vi "test Log Archive.vi"(8 "error in (no error)":errorcluster, 11 "TestCase in":refnum<class "Embedded Data Logger Windows System Tests.lvclass">) -> (0 "error out":errorcluster, 3 "TestCase out":refnum<class "Embedded Data Logger Windows System Tests.lvclass">)   [LabVIEW 2027, in "Embedded Data Logger Windows System Tests.lvclass"]
uses:
  Embedded Data Logger Windows System Tests.lvclass
  61a2513e-13d3-4fa2-bc23-ec2f6314a367.vi
  C:/Program Files/National Instruments/LabVIEW 2027/vi.lib/addons/_JKI Toolkits/VI Tester/TestCase.llb/TestCase.lvclass
  <vilib>/addons/_JKI Toolkits/VI Tester/TestCase.llb/TestCase.lvclass
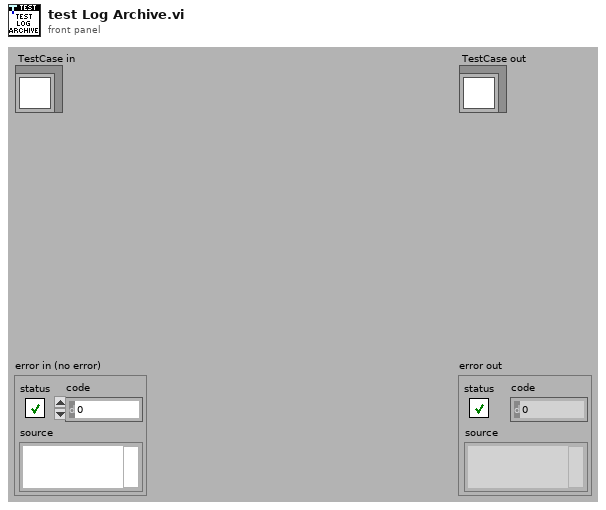
[diagram p1: front panel]
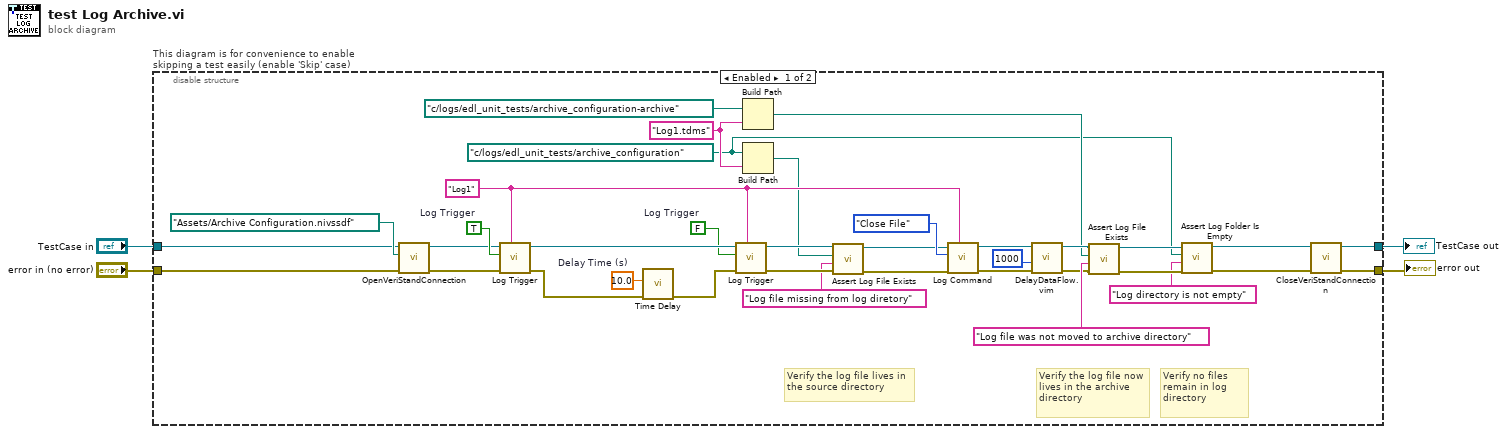
[diagram p0: block diagram]
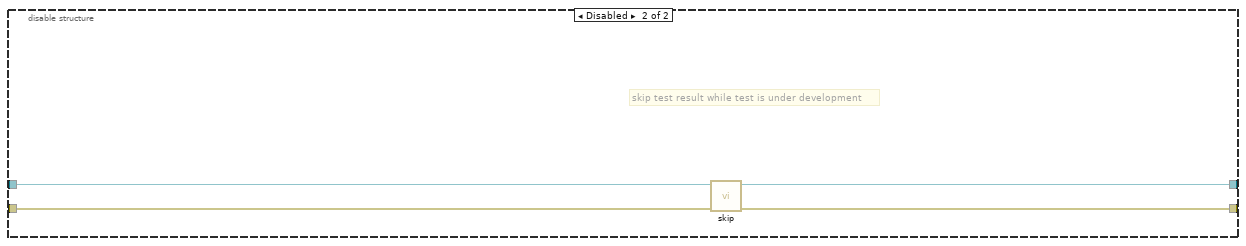
[diagram p2: hidden frame]
diagram:
  n1 = disable-structure "This diagram is for convenience to enable skipping a test easily (enable 'Skip' case)" shown="Enabled" {
    disable-tunnel: "TestCase in" -> [w13 w43]
    disable-tunnel: [w8 w41] -> w1
    disable-tunnel: [w9 w42] -> w3
    disable-tunnel: "error in (no error)" -> [w12 w40]
    frame Enabled {
      w22 = "Log1.tdms" ("Embedded Data Logger File Name")
      w19 = path "c:/logs/edl_unit_tests/archive_configuration" ("file path")
      w30 = "Log1" ("Embedded Data Logger File Name")
      w34 = FALSE  # Log Trigger
      w35 = 10.0  # Delay Time (s)
      w37 = TRUE  # Log Trigger
      # "Verify no files remain in log directory"
      # "Verify the log file now lives in the archive directory"
      # "Verify the log file lives in the source directory"
      n2 = call-dynamic "OpenVeriStandConnection.vi"("error in (no error)"=w12, "System Definition File"=path "Assets/Archive Configuration.nivssdf", "VeriStand Test Case in"=w13) -> ("error out"=w11:errorcluster, "VeriStand Test Case out"=w14:refnum<class "Embedded Data Logger Windows System Tests.lvclass">)  [unwired: 6 in, 1 out]
      n3 = call "Log Trigger.vi"("Embedded Data Logger File Name"=w30, "error in"=w11, "Log Trigger"=w37, "Embedded Data Logger System Tests in"=w14) -> ("error out"=w38:errorcluster, "Embedded Data Logger System Tests out"=w39:refnum<class "Embedded Data Logger Windows System Tests.lvclass">)  [unwired: 6 in]
      n4 = call "Time Delay"("error in (no error)"=w38, "Delay Time (s)"=w35) -> ("error out"=w36:errorcluster)  [unwired: 9 in]
      n5 = call "Log Trigger.vi"("Embedded Data Logger File Name"=w30, "error in"=w36, "Log Trigger"=w34, "Embedded Data Logger System Tests in"=w39) -> ("error out"=w28:errorcluster, "Embedded Data Logger System Tests out"=w29:refnum<class "Embedded Data Logger Windows System Tests.lvclass">)  [unwired: 6 in]
      n6 = Build Path(base path=path "c:/logs/edl_unit_tests/archive_configuration-archive" ("file path"), name or relative path=w22) -> (appended path=w20:path)
      n7 = Build Path(base path=w19, name or relative path=w22) -> (appended path=w21:path)
      n8 = call "Assert Log File Exists.vi"("error in"=w28, "message on error"="Log file missing from log diretory" ("message"), "file path"=w21, "Embedded Data Logger System Tests in"=w29) -> ("error out"=w26:errorcluster, "Embedded Data Logger System Tests out"=w27:refnum<class "Embedded Data Logger Windows System Tests.lvclass">)  [unwired: 6 in]
      n9 = call "Log Command.vi"("Embedded Data Logger File Name"=w30, "error in"=w26, "Log Command"=enum16{"Idle", "Open File", "Close File"}."Close File", "Embedded Data Logger System Tests in"=w27) -> ("error out"=w31:errorcluster, "Embedded Data Logger System Tests out"=w32:refnum<class "Embedded Data Logger Windows System Tests.lvclass">)  [unwired: 6 in]
      n10 = call "DelayDataFlow.vim"("value in"=w31, "milliseconds to wait"=u32 1000) -> ("value out"=w6:errorcluster)  [unwired: 2 in, 1 out]
      n11 = call "Assert Log File Exists.vi"("error in"=w6, "message on error"="Log file was not moved to archive directory" ("message"), "file path"=w20, "Embedded Data Logger System Tests in"=w32) -> ("error out"=w24:errorcluster, "Embedded Data Logger System Tests out"=w25:refnum<class "Embedded Data Logger Windows System Tests.lvclass">)  [unwired: 6 in]
      n12 = call "Assert Log Folder Is Empty.vi"("error in"=w24, "message on error"="Log directory is not empty" ("custom report message (\"\")"), "directory"=w19, "Embedded Data Logger System Tests in"=w25) -> ("error out"=w10:errorcluster, "Embedded Data Logger System Tests out"=w7:refnum<class "Embedded Data Logger Windows System Tests.lvclass">)  [unwired: 6 in]
      n13 = call-dynamic "CloseVeriStandConnection.vi"("error in (no error)"=w10, "VeriStand Test Case in"=w7) -> ("error out"=w9:errorcluster, "VeriStand Test Case out"=w8:refnum<class "Embedded Data Logger Windows System Tests.lvclass">)  [unwired: 8 in]
    }
    frame Disabled {
      # "skip test result while test is under development"
      n14 = call <vilib>:"skip.vi"("error in (no error)"=w40, "TestCase in"=w43) -> ("error out"=w42:errorcluster, "TestCase out"=w41:refnum<class "Embedded Data Logger Windows System Tests.lvclass">)  [unwired: 8 in]
    }
  }
  "error out" <- w3
  "TestCase out" <- w1
